vi "SQL_删除已有表.vi"(8 "error in (no error)":errorcluster caption="错误输入（无错误）", 10 "已有表名":string="d7") -> (0 "error out":errorcluster caption="错误输出", 3 "SQL_删除已有表":string)   [LabVIEW 2014]
doc: "该模板用于创建子VI。"
panel:
  # "varchar括号中的数值最大255"
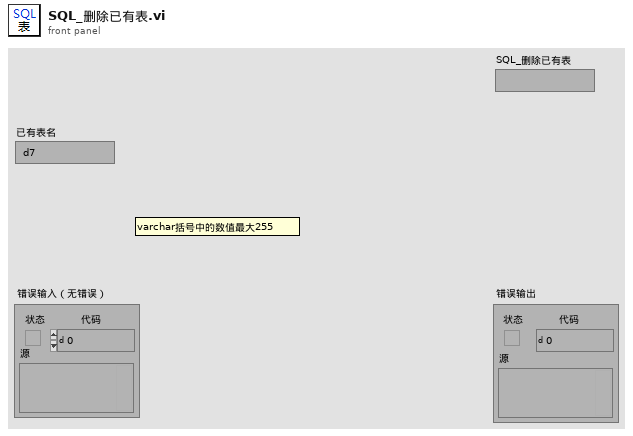
[diagram p1: front panel]
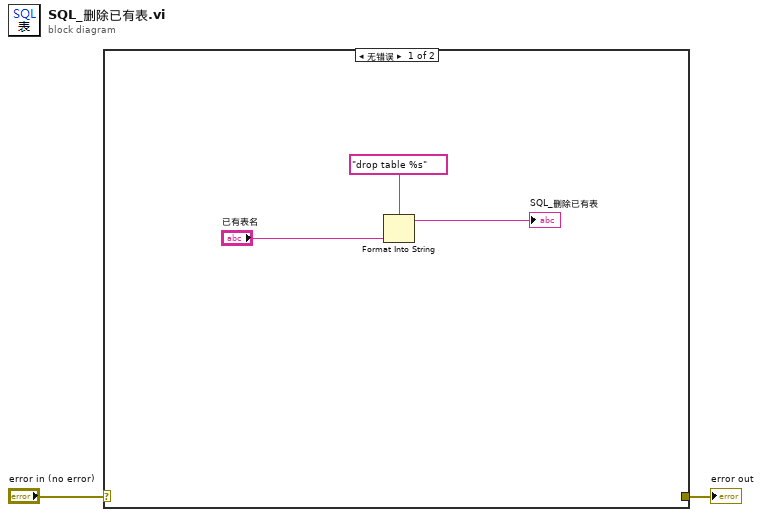
[diagram p0: block diagram]
diagram:
  n1 = case shown="无错误" "error in (no error)" {
    selector: "error in (no error)" -> [_ w6]
    tunnel: [_ w6] -> w1
    frame No Error {
      n2 = Format Into String(format string="drop table %s", "已有表名") -> (resulting string=→"SQL_删除已有表":string)  [unwired: 2 in, 1 out]
    }
    frame Error {
    }
  }
  "error out" <- w1
